vi "ConfigProgram2XML.vi"(8 "error in (no error)":errorcluster, 9 "Microscope":string[][](array[string]), 10 "Positions":string[][](array[string]), 11 "Program":string[][](array[string])) -> (0 "error out":errorcluster, 3 "ProgramPath":path)   [LabVIEW 2018, in "Config.lvlib"]
uses:
  Config.lvlib
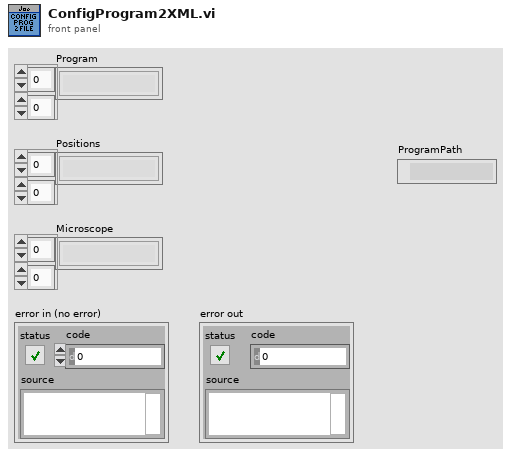
[diagram p1: front panel]
types:
  T1 = enum16{"open", "replace", "create", "open or create", "replace or create", "replace or create with confirmation"}
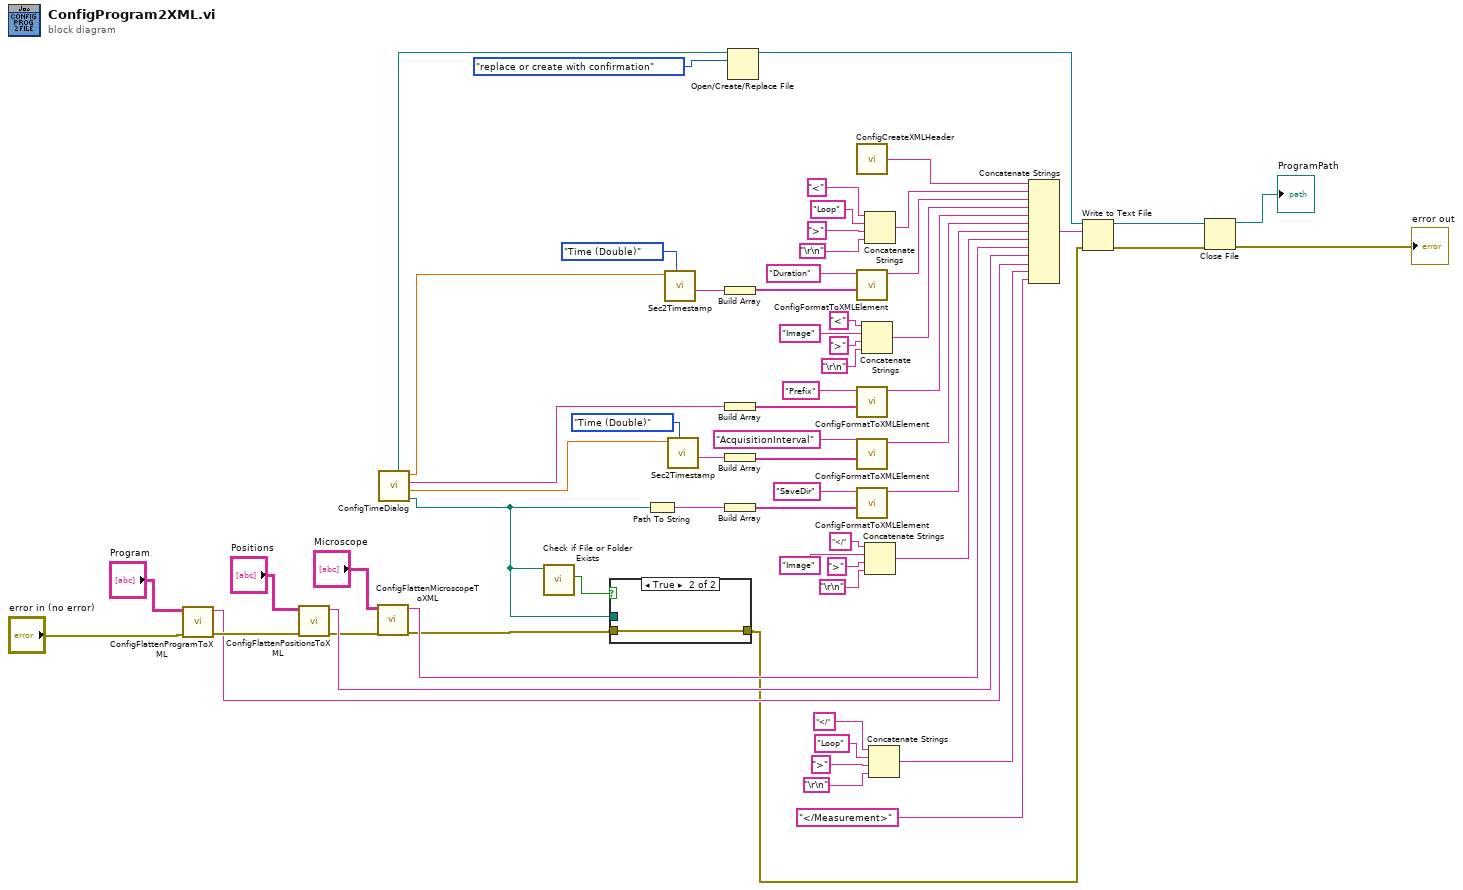
[diagram p0: block diagram]
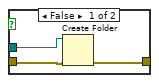
[diagram p2: hidden frame]
diagram:
  n1 = call "ConfigFlattenProgramToXML.vi"("error in (no error)"="error in (no error)", "ProgramArray"="Program") -> ("error out"=w57:errorcluster, "ProgramXML"=w55:string)  [unwired: 8 in]
  n2 = call "ConfigFlattenPositionsToXML.vi"("error in"=w57, "Position Array in"="Positions") -> ("error out"=w58:errorcluster, "Position XML"=w61:string)  [unwired: 8 in]
  n3 = call "ConfigFlattenMicroscopeToXML.vi"("error in (no error)"=w58, "MicroscopeArray"="Microscope") -> ("error out"=w10:errorcluster, "MicrosocopeXML"=w60:string)  [unwired: 8 in]
  n4 = call "ConfigTimeDialog.vi"() -> ("Image Folder out"=w6:path, "Interval out"=w7:dbl, "Prefix out"=w8:string, "Total out"=w9:dbl, "Config File Path"=w4:path)  [unwired: 7 in]
  n5 = call <vilib>:"Check if File or Folder Exists.vi"("path"=w6) -> ("file or folder exists?"=w5:bool)  [unwired: 8 in, 2 out]
  n6 = case shown="True" w5 {
    tunnel: w6 -> [w66 _]
    tunnel: [w65 w67] -> w11
    tunnel: w10 -> [w64 w67]
    frame False {
      n7 = Create Folder(path (use dialog)=w66, error in=w64) -> (error out=w65:errorcluster)  [unwired: 1 in, 2 out]
    }
    frame True {
    }
  }
  n8 = Path To String(path=w6) -> (string=w38:string)
  n9 = call "Sec2Timestamp.vi"("Input Selection"=enum32{"Time (Double)", "Time (Time Stamp)"}."Time (Double)", "Input Time (Double)"=w9) -> ("date/time string"=w47:string)  [unwired: 7 in, 2 out]
  n10 = call "Sec2Timestamp.vi"("Input Selection"=enum32{"Time (Double)", "Time (Time Stamp)"}."Time (Double)", "Input Time (Double)"=w7) -> ("date/time string"=w48:string)  [unwired: 7 in, 2 out]
  n11 = Build Array(w47) -> (w42:string[])
  n12 = Build Array(w8) -> (w35:string[])
  n13 = Build Array(w48) -> (w49:string[])
  n14 = Build Array(w38) -> (w39:string[])
  n15 = Open/Create/Replace File(file path (use dialog)=w4, operation (0:open)=T1."replace or create with confirmation") -> (refnum out=w3:refnum<file>)  [unwired: 4 in, 2 out]
  n16 = call "ConfigCreateXMLHeader.vi"() -> ("XML Header"=w51:string)
  n17 = call "ConfigFormatToXMLElement.vi"("Value"=w42, "outer Tag"="Duration" ("string")) -> ("Resulting String"=w43:string)  [unwired: 9 in]
  n18 = call "ConfigFormatToXMLElement.vi"("Value"=w35, "outer Tag"="Prefix" ("string")) -> ("Resulting String"=w36:string)  [unwired: 9 in]
  n19 = call "ConfigFormatToXMLElement.vi"("Value"=w49, "outer Tag"="AcquisitionInterval" ("string")) -> ("Resulting String"=w32:string)  [unwired: 9 in]
  n20 = call "ConfigFormatToXMLElement.vi"("Value"=w39, "outer Tag"="SaveDir" ("string")) -> ("Resulting String"=w40:string)  [unwired: 9 in]
  n21 = Concatenate Strings("<" ("string"), "Image" ("string"), ">" ("string"), "\r\n") -> (w21:string)
  n22 = Concatenate Strings("<" ("string"), "Loop" ("string"), ">" ("string"), "\r\n") -> (w25:string)
  n23 = Concatenate Strings("</" ("string"), "Image" ("string"), ">" ("string"), "\r\n") -> (w22:string)
  n24 = Concatenate Strings("</" ("string"), "Loop" ("string"), ">" ("string"), "\r\n") -> (w29:string)
  n25 = Concatenate Strings(w51, w25, w43, w21, w36, w32, w40, w22, w60, w61, w55, w29, "</Measurement>" ("string")) -> (w31:string)
  n26 = Write to Text File(file (use dialog)=w3, text=w31, error in=w11) -> (refnum out=w52:refnum<file>, error out=w53:errorcluster)  [unwired: 1 in, 1 out]
  n27 = Close File(refnum=w52, error in=w53) -> (path=→"ProgramPath":path, error out=→"error out":errorcluster)
